vi "SequenceRunReference.vi"(5 "EndTime":timestamp, 7 "StartTime":timestamp, 8 "error in":errorcluster, 11 "Defect":refnum<class "SequenceRunReference.lvclass">) -> (0 "error out":errorcluster, 3 "Passed":bool)   [LabVIEW 2020]
uses:
  ProligentResultProcessor/Failure/FailureReference/SetId.vi
  ProligentResultProcessor/Failure/FailureReference/GetId.vi
  ProligentResultProcessor/Failure/FailureReference/GetCustomData.vi
  ProligentResultProcessor/Model/CustomData/CustomData.lvclass
  ProligentResultProcessor/SequenceRun/SequenceRunReference/SequenceRunReference.lvclass
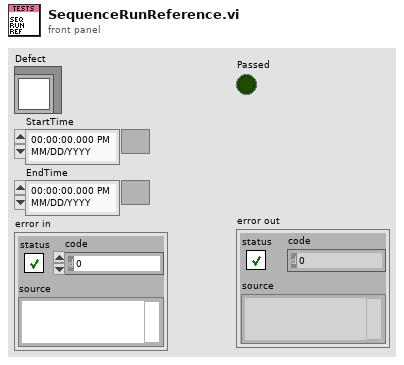
[diagram p1: front panel]
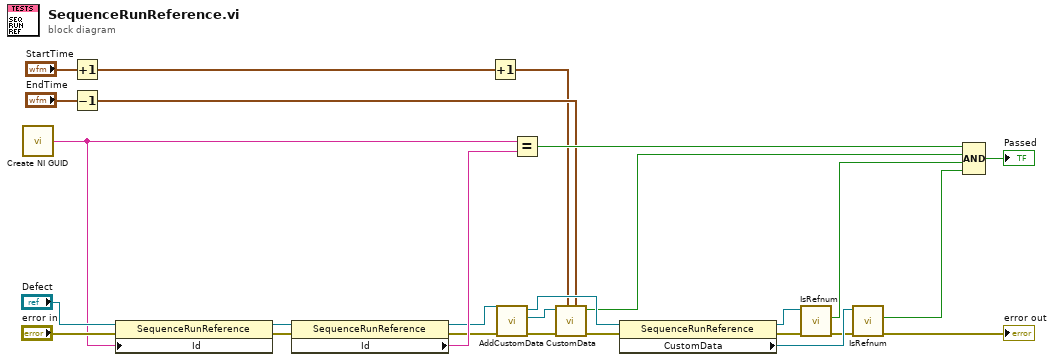
[diagram p0: block diagram]
diagram:
  n1 = call <vilib>:"Create NI GUID.vi"() -> ("NI GUID"=w1:string)
  n2 = Increment(x="StartTime") -> (x+1=w5:timestamp)
  n3 = Decrement(x="EndTime") -> (x-1=w6:timestamp)
  n4 = property class="SequenceRunReference"(reference="Defect", error in="error in", "Id"=w1) -> (reference out=w25:refnum<class "SequenceRunReference.lvclass">, error out=w24:errorcluster)
  n5 = property class="SequenceRunReference"(reference=w25, error in=w24) -> (reference out=w2:refnum<class "SequenceRunReference.lvclass">, error out=w3:errorcluster, "Id"=w23:string)
  n6 = Increment(x=w5) -> (x+1=w4:timestamp)
  n7 = call "AddCustomData.vi"("error in"=w3, "SequenceRunReference in"=w2) -> ("error out"=w14:errorcluster, "CustomData"=w13:refnum<class "CustomData.lvclass">, "SequenceRunReference out"=w15:refnum<class "SequenceRunReference.lvclass">)  [unwired: 7 in]
  n8 = Equal?(x=w1, y=w23) -> (x = y?=w21:bool)
  n9 = call "CustomData.vi"("EndTime"=w6, "StartTime"=w4, "error in"=w14, "CustomData"=w13) -> ("error out"=w12:errorcluster, "Passed"=w7:bool)  [unwired: 6 in]
  n10 = property class="SequenceRunReference"(reference=w15, error in=w12) -> (reference out=w17:refnum<class "SequenceRunReference.lvclass">, error out=w22:errorcluster, "CustomData"=w11:refnum<class "CustomData.lvclass">)
  n11 = call "IsRefnum.vi"("error in"=w22, "SequenceRunReference in"=w17) -> ("error out"=w10:errorcluster, "IsRefnum"=w16:bool)  [unwired: 7 in, 1 out]
  n12 = call "IsRefnum.vi"("error in"=w10, "CustomDataType in"=w11) -> ("error out"=→"error out":errorcluster, "IsRefnum"=w8:bool)  [unwired: 7 in, 1 out]
  n13 = Compound Arithmetic op=AND(w21, w7, w16, w8) -> (→"Passed":bool)
